vi "Config Process.vi"(8 "error in (no error)":errorcluster, 11 "View Model":T1) -> (0 "error out":errorcluster)   [LabVIEW 2017]
doc: "Provides interface for processing all operations with Configuration DB.\n[Covers: CD5]"
uses:
  View Model/Controls/View Model.ctl
  View Model/Controls/Shared Model.ctl
  Error Handler/Controls/Error Model.ctl
  Error Handler/Controls/Error Data.ctl
  Error Handler/Controls/Error Type.ctl
  Error Handler/Controls/Error Source.ctl
  Controls/Config Model.ctl
  Controls/Config CMD.ctl
  Controls/Config Command.ctl
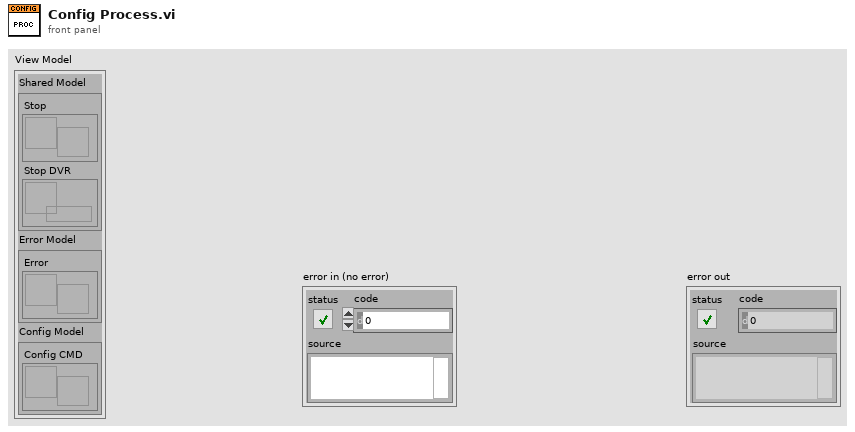
[diagram p1: front panel]
types:
  T1 = typedef "View Model.ctl" = cluster{"Shared Model":T2, "Error Model":T3, "Config Model":T4}
  T2 = typedef "Shared Model.ctl" = cluster{"Stop":refnum<user-event>, "Stop DVR":refnum<data-value>}
  T3 = typedef "Error Model.ctl" = cluster{"Error":refnum<user-event>}
  T4 = typedef "Config Model.ctl" = cluster{"Config CMD":refnum<user-event>}
  T5 = typedef "Config Command.ctl" = enum16{"Read", "Search", "Update"}
  T6 = typedef "Config Data Record.ctl" = cluster{"Account Number":u32, "First Name":string, "Last Name":string, "Balance":dbl}
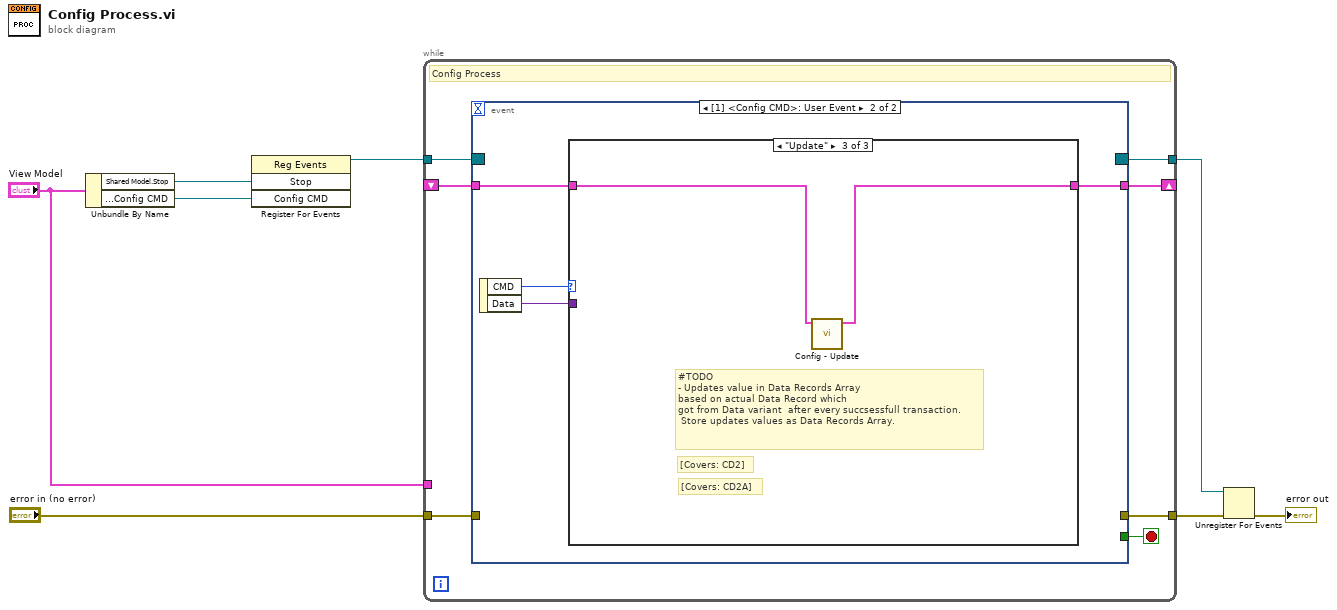
[diagram p0: block diagram]
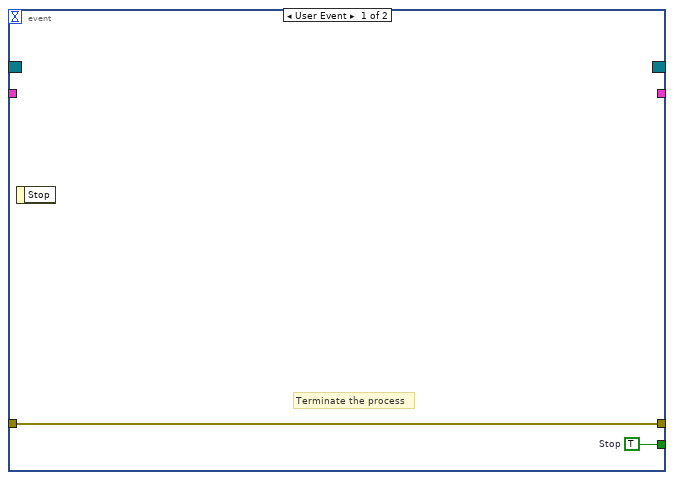
[diagram p2: hidden frame]
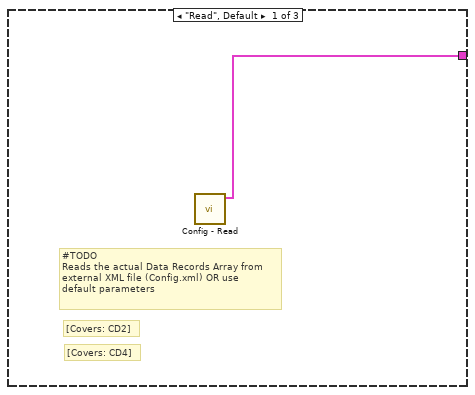
[diagram p3: hidden frame]
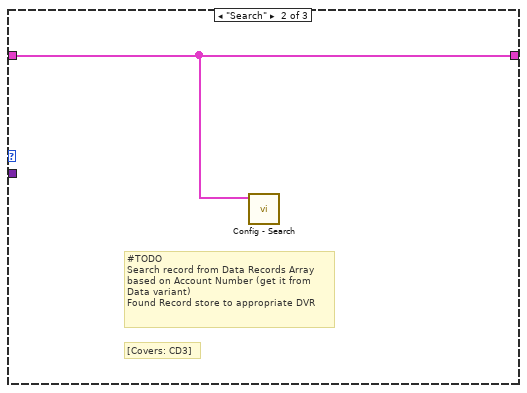
[diagram p4: hidden frame]
diagram:
  n1 = Unbundle By Name("View Model") -> ("Shared Model.Stop"=w8:refnum<user-event>, "Config Model.Config CMD"=w1:refnum<user-event>)
  n2 = register-events(w8, w1) -> (reference out=w7:refnum<event-registration>)  [unwired: 2 in, 1 out]
  n3 = while {
    tunnel: w7 -> [w15]
    tunnel: [w14] -> w6
    tunnel: "error in (no error)" -> [w13]
    tunnel: [w12] -> w3
    tunnel: "View Model" -> [_]
    shift-right: [w10] -> _
    shift-left: _ -> [w9]
    stop <- w11 stop-if-true
    # "Config Process"
    n4 = event shown="[1] <Config CMD>: User Event" {
      selector: w15 -> [_ _]
      dyn-events: [_ _] -> w14
      timeout: _ -> [_ _]
      tunnel: w13 -> [w17 _]
      tunnel: [w17 _] -> w12
      tunnel: [w16 _] -> w11
      tunnel: [_ w19] -> w10
      tunnel: w9 -> [_ w18]
      event User Event {
        w16 = TRUE  # Stop
        # "Terminate the process"
        n5 = event-data() -> ()  [unwired: 1 in, 1 out]
      }
      event User Event {
        n6 = event-data() -> ("CMD"=w21:T5, "Data"=w20:variant)  [unwired: 1 in]
        n7 = case shown="\"Update\"" w21 {
          tunnel: w20 -> [_ _ _]
          tunnel: [w22 w23 w24] -> w19
          tunnel: w18 -> [_ w23 w25]
          frame "Read", Default {
            # "[Covers: CD4]"
            # "[Covers: CD2]"
            # "#TODO\nReads the actual Data Records Array from\nexternal XML file (Config.xml) OR use \ndefault parameters"
            n8 = call "Config - Read.vi"() -> ("Data Records"=w22:T6[])  [unwired: 10 in, 1 out]
          }
          frame "Search" {
            # "[Covers: CD3]"
            # "#TODO\nSearch record from Data Records Array\nbased on Account Number (get it from\nData variant)\nFound Record store to appropriate DVR"
            n9 = call "Config - Search.vi"("Data Records"=w23) -> ()  [unwired: 9 in, 2 out]
          }
          frame "Update" {
            # "[Covers: CD2A]"
            # "[Covers: CD2]"
            # "#TODO\n- Updates value in Data Records Array\nbased on actual Data Record which\ngot from Data variant  after every succsessfull transaction.\n Store updates values as Data Records Array."
            n10 = call "Config - Update.vi"("Data Records"=w25) -> ("Data Records"=w24:T6[])  [unwired: 9 in, 1 out]
          }
        }
      }
    }
  }
  n11 = Unregister For Events(event registration refnum=w6, error in=w3) -> (error out=→"error out":errorcluster)
